vi "Select Patch.vi"(4 "error in (no error)":errorcluster, 5 "patch?":i32, 6 "channel":i32, 7 "MIDI out handle":i32) -> (0 "error out":errorcluster, 1 "Win32 error code":i32, 3 "duplicate MIDI handle":i32)   [LabVIEW 2014]
doc: "Sends the MIDI Voice and MIDI Channel information to the MIDI Output Device my means of a MIDI Short Message."
panel:
  # "Input Data"
  # "Local Data"
  # "Output Data"
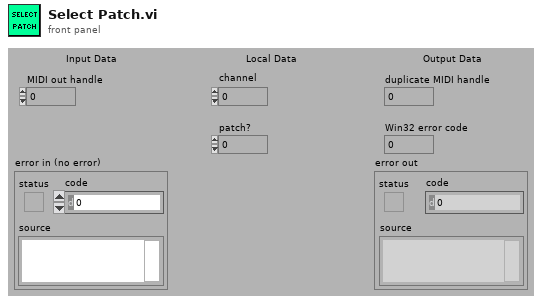
[diagram p1: front panel]
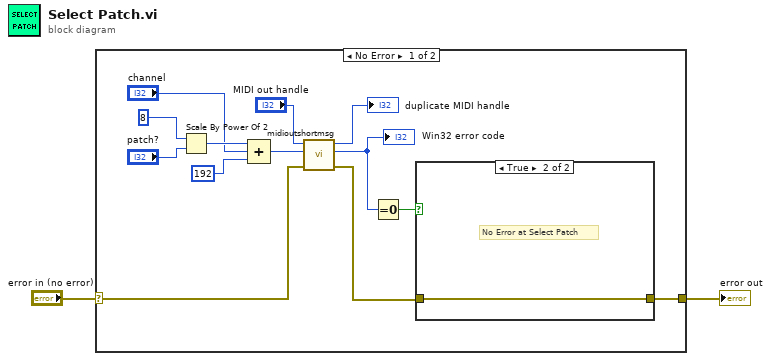
[diagram p0: block diagram]
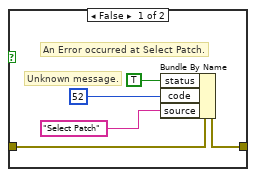
[diagram p2: hidden frame]
diagram:
  n1 = case shown="No Error" "error in (no error)" {
    selector: "error in (no error)" -> [w4 w22]
    tunnel: [w10 w22] -> w1
    frame No Error {
      n2 = Scale By Power Of 2(n=8, x="patch?") -> (x*2^n=w15:i32)
      n3 = Compound Arithmetic op=ADD(w15, "channel", 192 ("data")) -> (w7:i32)
      n4 = call "midioutshortmsg.vi"("error in (no error)"=w4, "data"=w7, "MIDI output handle"="MIDI out handle") -> ("error out"=w3:errorcluster, "Win32 error code"=w5:i32, "duplicate MIDI output handle"=→"duplicate MIDI handle":i32)  [unwired: 2 in]
      "Win32 error code" <- w5
      n5 = Equal To 0?(x=w5) -> (x = 0?=w9:bool)
      n6 = case shown="True" w9 {
        tunnel: w3 -> [w20 w21]
        tunnel: [w19 w21] -> w10
        frame False {
          # "Unknown message."
          # "An Error occurred at Select Patch."
          n7 = Bundle By Name(cluster=w20, "status"=TRUE, "code"=52, "source"="Select Patch") -> (w19:errorcluster)
        }
        frame True {
          # "No Error at Select Patch"
        }
      }
    }
    frame Error {
    }
  }
  "error out" <- w1
